vi "Client_Initialization.vi"(8 "error in (no error)":errorcluster, 11 "Modeli.lvlib:Modeli.lvclass":refnum<class "Modeli.lvclass">) -> (0 "error out":errorcluster, 2 "Event Registration Refnum":refnum<event-registration>, 3 "Modeli.lvlib:Modeli.lvclass 2":refnum<class "Modeli.lvclass">)   [LabVIEW 2018, in "Modeli.lvlib" / "Modeli.lvclass"]
uses:
  Modeli.lvclass
  Modeli.lvclass/Modeli.ctl
  Projects/PRJ-Quasar Listening/Quasar Listening/x64/Release/Quasar Listening.dll
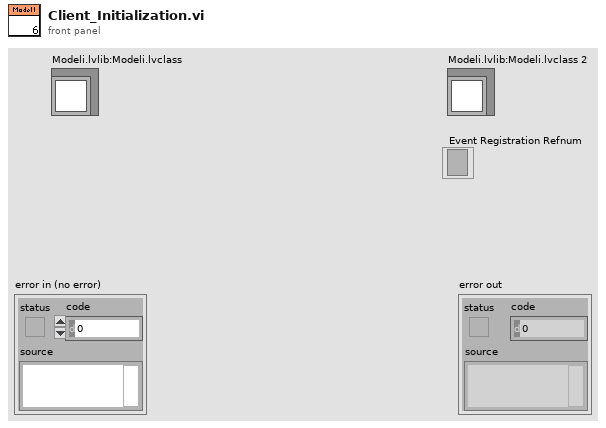
[diagram p1: front panel]
types:
  T1 = cluster{"points":u64, "intensity":u16, "azimuth":dbl, "elevation":dbl, "range":dbl, "site":u8}
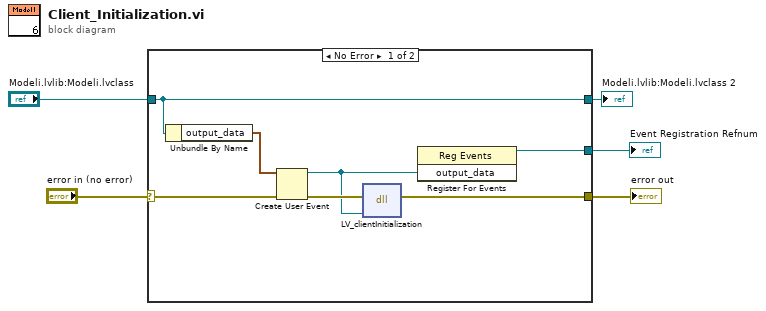
[diagram p0: block diagram]
diagram:
  n1 = case shown="No Error" "error in (no error)" {
    selector: "error in (no error)" -> [w11 w14]
    tunnel: [w12 w14] -> w4
    tunnel: "Modeli.lvlib:Modeli.lvclass" -> [w6 w13]
    tunnel: [w7 _] -> w3
    tunnel: [w6 w13] -> w2
    frame No Error {
      n2 = Unbundle By Name(w6) -> ("output_data"=w9:T1)
      n3 = Create User Event(user event datatype=w9, error in=w11) -> (user event=w8:refnum<user-event>, error out=w10:errorcluster)
      n4 = dll-call lib="C:/Projects/PRJ-Quasar Listening/Quasar Listening/x64/Release/Quasar Listening.dll" fn="LV_clientInitialization"(error in=w10, "refnum"=w8) -> (error out=w12:errorcluster)  [unwired: 4 in, 1 out]
      n5 = register-events(w8) -> (reference out=w7:refnum<event-registration>)  [unwired: 2 in, 1 out]
    }
    frame Error {
    }
  }
  "error out" <- w4
  "Event Registration Refnum" <- w3
  "Modeli.lvlib:Modeli.lvclass 2" <- w2
